vi "DB5000.R读取.vi"(0 "gInitialSIEMENSS7 In":refnum<k24>, 1 "地址数组":string[](array[string])=["DB5000.136", "DB5000.140", "DB5000.144", "DB5000.148", "DB5000.152", "DB5000.156", "DB5000.160", "DB5000.164", "DB5000.168", "DB5000.172", "DB5000.176"], 5 "error in (no error)":errorcluster caption="错误输入（无错误）") -> (14 "gInitialSIEMENSS7 Out":refnum<k24>, 15 "IsSuccess":bool, 17 "添加的数组":sgl[](array[numeric]), 18 "DB5000.R":T1, 19 "error out":errorcluster caption="错误输出")   [LabVIEW 2017]
panel:
  # "DB5000,REAL136"
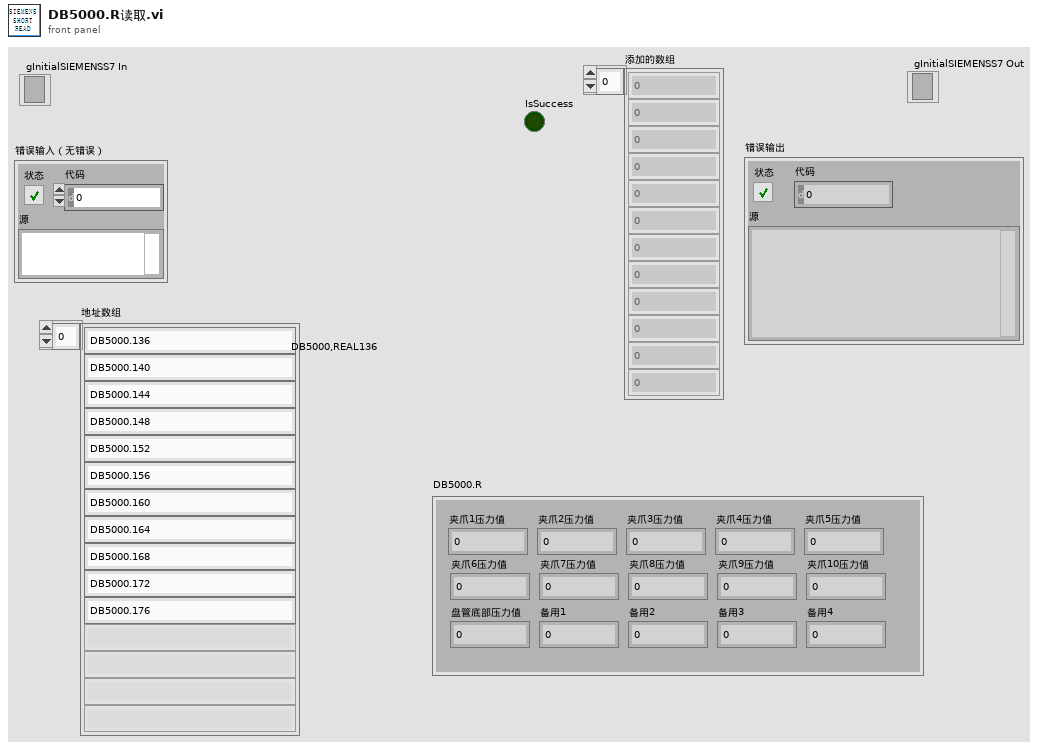
[diagram p1: front panel]
types:
  T1 = cluster{"夹爪1压力值":sgl, "夹爪2压力值":sgl, "夹爪3压力值":sgl, "夹爪4压力值":sgl, "夹爪5压力值":sgl, "夹爪6压力值":sgl, "夹爪7压力值":sgl, "夹爪8压力值":sgl, "夹爪9压力值":sgl, "夹爪10压力值":sgl, "盘管底部压力值":sgl, "备用1":sgl, "备用2":sgl, "备用3":sgl, "备用4":sgl}
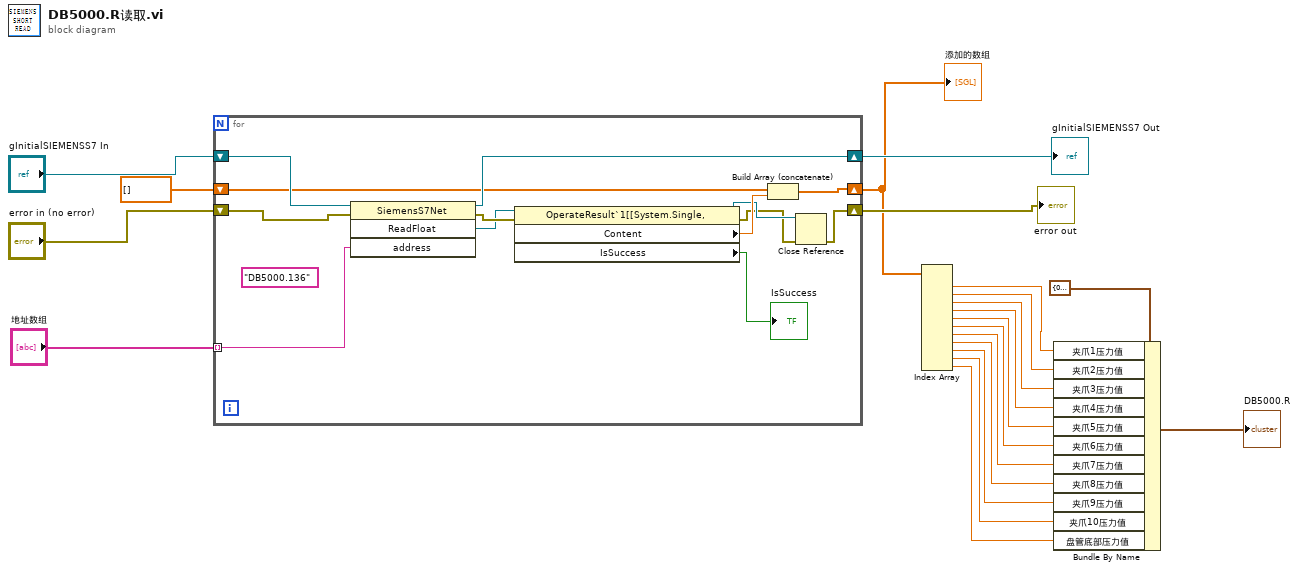
[diagram p0: block diagram]
diagram:
  n1 = for {
    shift-right: [w29] -> w17
    shift-left: "gInitialSIEMENSS7 In" -> [w33]
    shift-right: [w21] -> w18
    shift-left: "error in (no error)" -> [w32]
    tunnel: "地址数组" -> [w28] mode=indexing
    shift-right: [w25] -> w14
    shift-left: sgl[] [] ("添加的数组") -> [w26]
    (unwired) "DB5000.136" ("address")
    n2 = invoke class="SiemensS7Net" method="ReadFloat"(reference=w33, error in=w32, "address"=w28) -> (reference out=w29:refnum<k24>, error out=w31:errorcluster, "ReadFloat"=w30:refnum<k24>)  [unwired: 1 in, 1 out]
    n3 = property class="OperateResult`1[[System.Single,"(reference=w30, error in=w31) -> (reference out=w23:refnum<k24>, error out=w22:errorcluster, "Content"=w27:sgl, "IsSuccess"=→"IsSuccess":bool)
    n4 = Build Array (concatenate)(w26, w27) -> (w25:sgl[])
    n5 = Close Reference(reference=w23, error in (no error)=w22) -> (error out=w21:errorcluster)
  }
  "gInitialSIEMENSS7 Out" <- w17
  "error out" <- w18
  "添加的数组" <- w14
  n6 = Index Array(array=w14) -> (element #1=w11:sgl, element #2=w10:sgl, element #3=w9:sgl, element #4=w8:sgl, element #5=w7:sgl, element #6=w6:sgl, element #7=w5:sgl, element #8=w4:sgl, element #9=w3:sgl, element #10=w2:sgl, element #11=w1:sgl)  [unwired: 11 in]
  n7 = Bundle By Name(cluster=T1 {"夹爪1压力值"=0.0, "夹爪2压力值"=0.0, "夹爪3压力值"=0.0, "夹爪4压力值"=0.0, "夹爪5压力值"=0.0, "夹爪6压力值"=0.0, "夹爪7压力值"=0.0, "夹爪8压力值"=0.0, "夹爪9压力值"=0.0, "夹爪10压力值"=0.0, "盘管底部压力值"=0.0, "备用1"=0.0, "备用2"=0.0, "备用3"=0.0, "备用4"=0.0} ("DB5000.R"), "夹爪1压力值"=w11, "夹爪2压力值"=w10, "夹爪3压力值"=w9, "夹爪4压力值"=w8, "夹爪5压力值"=w7, "夹爪6压力值"=w6, "夹爪7压力值"=w5, "夹爪8压力值"=w4, "夹爪9压力值"=w3, "夹爪10压力值"=w2, "盘管底部压力值"=w1) -> (→"DB5000.R":T1)
